vi "EXAMPLE - Determine Clicked Array Element Index.vi"() -> ()   [LabVIEW 2016]
doc: "EXAMPLE - Determine Clicked Array Element Index.vi\n\nDescription:\nThis example VI deomonstrates how to use the Determine Clicked Array Element Index VI to determine the index of the array element clicked by a user.\n\nThe VI returns the correct index whether:\n- the array is a 1D or 2D array\n- the array is displayed horizontally or vertically\n- the array label, caption, scrollbars or index display are visible or not\n- the array has an element gap displayed\n- the array array elements are physically large or small\n- the user has scrolled the visible portion of the array using either the index controls or the scrollbars\n\nNOTE: Proper operation of the Determine Clicked Array Element Index VI requires that a caption has been created for the array of interest by following the numbered steps below:\n\n(1) Right click on the array of interest and select Visible Items >> Caption\n(The item should be checked)\n\n(2) Right click on the array of interest and select Visible Items >> Caption\n(The item should be un-checked)\n\n(3) Right click on the array of interest and select Visible Items >> Label\n(The item should be checked)\n\n(4) Save the VI\n\nDeveloped By:\nMark.ridgley\nMark.Ridgley_LabVIEW.Developer@comcast.net"
panel:
  in  "stop":bool
  out "Clicked Index":i32[](array[numeric])
  in  "Tab Control":T1(tab)
  out "2D Array (With element gap)":picture[][](array[picture]) caption="2D Array"
  out "2D Array":picture[][](array[picture])
  out "2D Array of Small Elements (With elemet gap)":picture[][](array[picture])
  out "2D Array of Small Elements":picture[][](array[picture])
  out "1D Array (Vertical with elemet gap)":picture[](array[picture])
  out "1D Array (Vertical)":picture[](array[picture])
  out "1D Array (Horizontal with element gap)":picture[](array[picture])
  out "1D Array (Horizontal)":picture[](array[picture])
  out "Selected Glyph":picture
  out "Array of Glyphs":picture[][](array[picture])
  out "Selected Element":string
  out "2D Array of Strings (With element gap)":string[][](array[string]) caption="2D Array"
  # "Run the VI. Click an element in any array on any tab.\n\nThe clicked index indicator will display the index of the element you clicked.\n\nThe VI returns the correct index whether:\n- the array is a 1D or 2D array\n- the array is displayed horizontally or vertically\n- the array label, caption, scrollbars or index display are visible or not\n- the array has an element gap displayed\n- the array array elements are physically large or small\n- the user has scrolled the visible portion of the array using either the index controls or the scrollbars"
  # "Row"
  # "Col"
  # "This tab demonstrates how you can use the Determine Clicked Array Element Index VI to create an interface that is similar to the glyph selector in the NI Icon Editor."
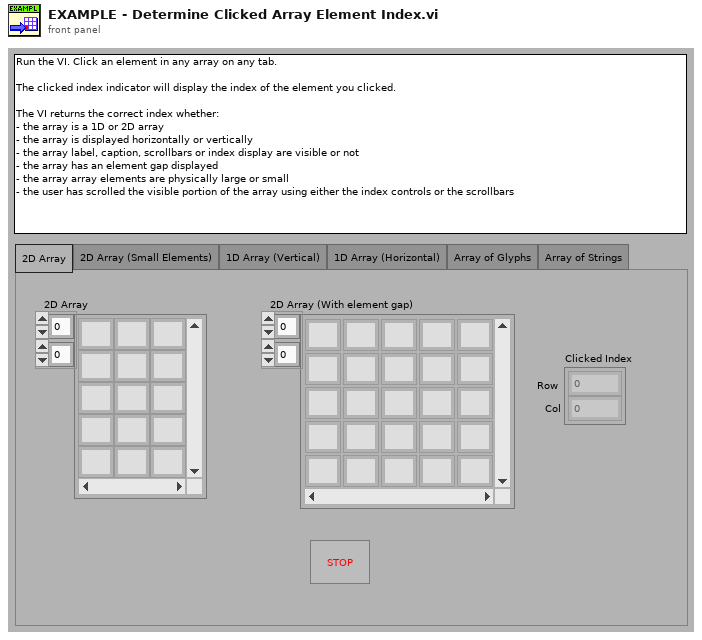
[diagram p1: front panel]
types:
  T1 = enum32{"2D Array", "2D Array (Small Elements)", "1D Array (Vertical)", "1D Array (Horizontal)", "Array of Glyphs", "Array of Strings"}
  T2 = typedef "imagedata.ctl" = cluster{"image type":i32, "image depth":i32, "image":u8[], "mask":u8[], "colors":u32[], "Rectangle":cluster{"left":i16, "top":i16, "right":i16, "bottom":i16}}
  T3 = typedef "LVPoint32TypeDef.ctl" = cluster{"Horizontal":i32, "Vertical":i32}
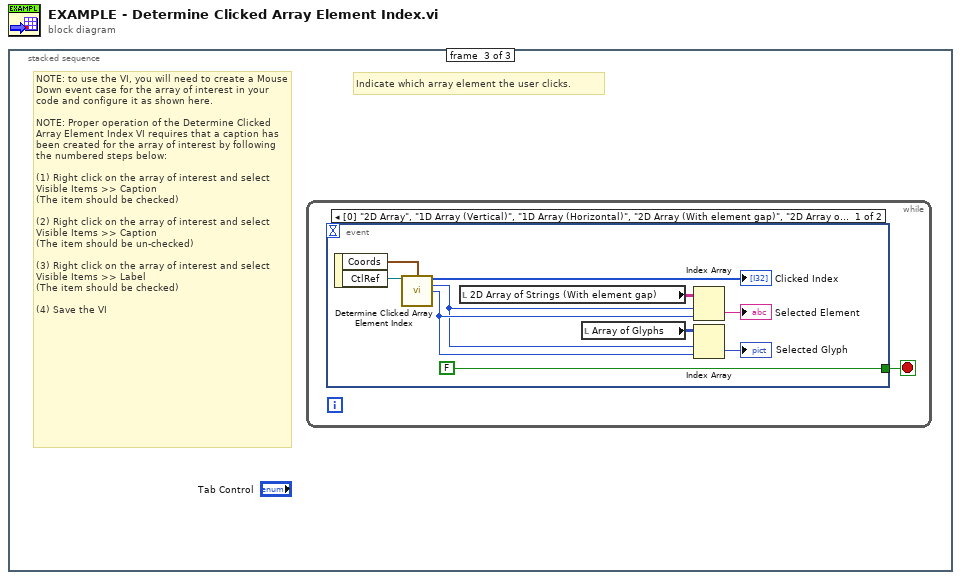
[diagram p0: block diagram]
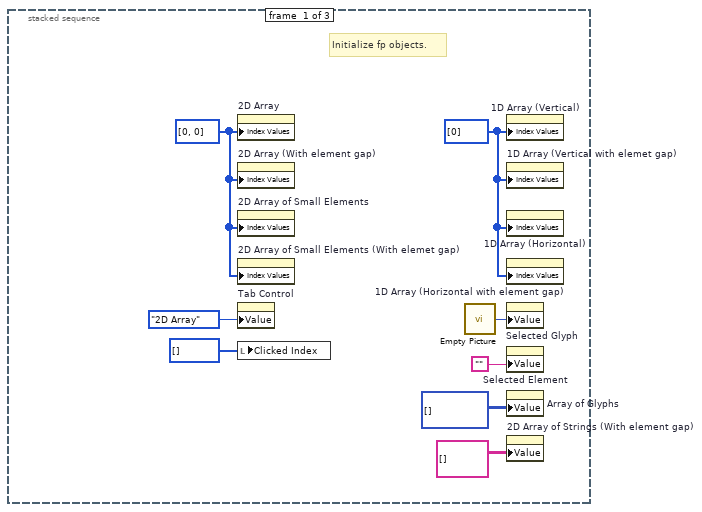
[diagram p2: hidden frame]
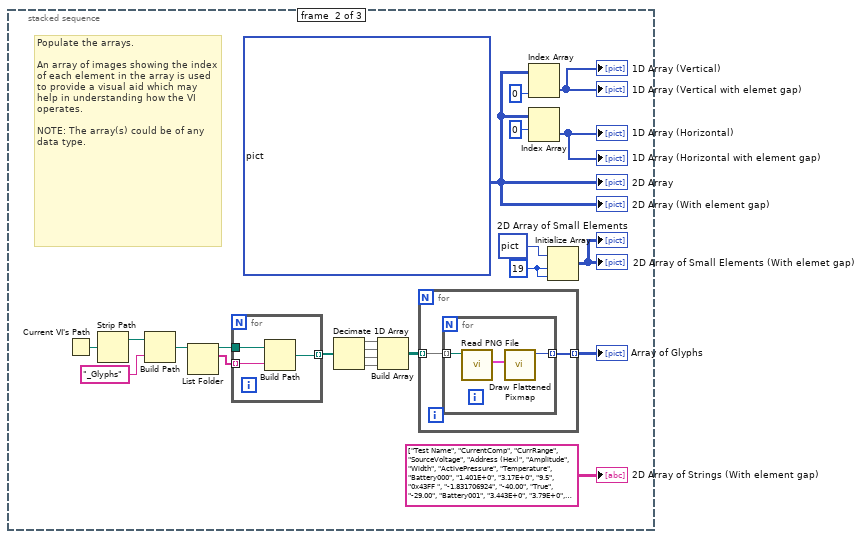
[diagram p3: hidden frame]
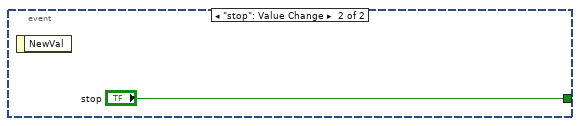
[diagram p4: hidden frame]
diagram:
  n1 = stacked-sequence {
    frame #0 {
      w6 = u32[] [0] ("Index Values")
      w7 = u32[] [0, 0] ("Selection Size[]")
      # "Initialize fp objects."
      n2 = property on="2D Array" class="Arr (strict)"("Index Values"=w7) -> ()  [unwired: 2 in, 2 out]
      n3 = property on="2D Array (With element gap)" class="Arr (strict)"("Index Values"=w7) -> ()  [unwired: 2 in, 2 out]
      n4 = property on="2D Array of Small Elements" class="Arr (strict)"("Index Values"=w7) -> ()  [unwired: 2 in, 2 out]
      n5 = property on="2D Array of Small Elements (With elemet gap)" class="Arr (strict)"("Index Values"=w7) -> ()  [unwired: 2 in, 2 out]
      n6 = property on="Tab Control" class="TabCtl (strict)"("Value"=T1."2D Array" ("Tab Control")) -> ()  [unwired: 2 in, 2 out]
      n7 = local write "Clicked Index"(i32[] [] ("Clicked Index")) -> ()
      n8 = call "Empty Picture"() -> ("empty picture"=w4:picture)
      n9 = property on="1D Array (Vertical)" class="Arr (strict)"("Index Values"=w6) -> ()  [unwired: 2 in, 2 out]
      n10 = property on="1D Array (Vertical with elemet gap)" class="Arr (strict)"("Index Values"=w6) -> ()  [unwired: 2 in, 2 out]
      n11 = property on="1D Array (Horizontal)" class="Arr (strict)"("Index Values"=w6) -> ()  [unwired: 2 in, 2 out]
      n12 = property on="1D Array (Horizontal with element gap)" class="Arr (strict)"("Index Values"=w6) -> ()  [unwired: 2 in, 2 out]
      n13 = property on="Selected Glyph" class="Pict"("Value"=w4) -> ()  [unwired: 2 in, 2 out]
      n14 = property on="Selected Element" class="Str"("Value"="") -> ()  [unwired: 2 in, 2 out]
      n15 = property on="Array of Glyphs" class="Arr (strict)"("Value"=picture[][] [] ("Array of Glyphs")) -> ()  [unwired: 2 in, 2 out]
      n16 = property on="2D Array of Strings (With element gap)" class="Arr (strict)"("Value"=string[][] [] ("2D Array of Strings (With element gap)")) -> ()  [unwired: 2 in, 2 out]
    }
    frame #1 {
      w27 = 19 ("dimension size")
      w26 = picture[][] [[bytes[3102], bytes[3102], bytes[3102], bytes[3102], bytes[3102]], [bytes[3102], bytes[3102], bytes[3102], bytes[3102], bytes[3102]], [bytes[3102], bytes[3102], bytes[3102], bytes[3102], bytes[3102]], [bytes[3102], bytes[3102], bytes[3102], bytes[3102], bytes[3102]], [bytes[3102], bytes[3102], bytes[3102], bytes[3102], bytes[3102]], [bytes[3102], bytes[3102], bytes[3102], bytes[3102], bytes[3102]], [bytes[3102], bytes[3102], bytes[3102], bytes[3102], bytes[3102]]] ("Array")
      # "Populate the arrays.\n\nAn array of images showing the index of each element in the array is used to provide a visual aid which may help in understanding how the VI operates.\n\nNOTE: The array(s) could be of any data type."
      n17 = Current VI's Path() -> (path=w10:path)
      n18 = Strip Path(path=w10) -> (stripped path=w11:path)  [unwired: 1 out]
      n19 = Build Path(base path=w11, name or relative path="_Glyphs") -> (appended path=w13:path)
      n20 = List Folder(path=w13) -> (path out=w22:path, filenames=w21:string[])  [unwired: 3 in, 2 out]
      n21 = for {
        tunnel: w22 -> [w33]
        tunnel: w21 -> [w32] mode=indexing
        tunnel: [w31] -> w20 mode=indexing
        n22 = Build Path(base path=w33, name or relative path=w32) -> (appended path=w31:path)
      }
      n23 = Decimate 1D Array(w20) -> (w19:path[], w18:path[], w17:path[], w16:path[])
      n24 = Build Array(w19, w18, w17, w16) -> (w15:path[][])
      n25 = for {
        tunnel: w15 -> [w35] mode=indexing
        tunnel: [w34] -> w14 mode=indexing
        n26 = for {
          tunnel: w35 -> [w37] mode=indexing
          tunnel: [w36] -> w34 mode=indexing
          n27 = call <vilib>:"Read PNG File.vi"("path to PNG file"=w37) -> ("image data"=w38:T2)  [unwired: 8 in, 2 out]
          n28 = call <vilib>:"Draw Flattened Pixmap.vi"("image data"=w38) -> ("new picture"=w36:picture)  [unwired: 8 in]
        }
      }
      "Array of Glyphs" <- w14
      n29 = Index Array(array=w26, index (col)=0 ("index (row)")) -> (element=→"1D Array (Vertical)" →"1D Array (Vertical with elemet gap)":picture[])  [unwired: 1 in]
      n30 = Index Array(array=w26, index (row)=0) -> (element=→"1D Array (Horizontal)" →"1D Array (Horizontal with element gap)":picture[])  [unwired: 1 in]
      n31 = Initialize Array(picture bytes[3102] ("Source Icon 2"), w27, w27) -> (→"2D Array of Small Elements" →"2D Array of Small Elements (With elemet gap)":picture[][])
      "2D Array" <- w26
      "2D Array (With element gap)" <- w26
      "2D Array of Strings (With element gap)" <- string[][] [["Test Name", "CurrentComp", "CurrRange", "SourceVoltage", "Address (Hex)", "Amplitude", "Width", "ActivePressure", "Temperature"], ["Battery000", "1.401E+0", "3.17E+0", "9.5", "0x43FF ", "-1.831706924", "-40.00", "True", "-29.00"], ["Battery001", "3.443E+0", "3.79E+0", "12", "0x7740 ", "3.258019614", "20.00", "False", "12.00"], ["Battery002", "1.234E+0", "3.79E+0", "12", "0x0896 ", "1.482121841", "10.00", "True", "1.00"], ["Battery003", "5.058E-1", "3.54E-1", "2.8", "0x7F5D ", "0.218707632", "40.00", "False", "26.00"], ["Battery004", "3.576E+0", "2.40E+0", "5.0", "0x4C5D ", "1.896321814", "50.00", "True", "33.00"], ["Battery005", "2.621E+0", "3.96E+0", "12", "0x597E ", "-3.832147003", "-50.00", "False", "-37.00"], ["Battery006", "3.412E+0", "1.21E+0", "3.2", "0x9157 ", "3.655155688", "50.00", "True", "36.00"], ["Battery007", "1.892E-1", "2.05E+0", "5.0", "0xC4F4 ", "0.418100465", "50.00", "False", "33.00"], ["Battery008", "2.545E+0", "1.76E+0", "5.0", "0x4104 ", "1.217330504", "20.00", "True", "9.00"], ["Battery009", "2.001E+0", "1.25E+0", "3.2", "0x63E6 ", "0.527299613", "40.00", "False", "27.00"], ["Battery010", "3.321E+0", "8.32E-1", "3.2", "0x1037 ", "2.886781355", "20.00", "True", "9.00"], ["Battery011", "1.465E-1", "3.86E+0", "12", "0xB6C7 ", "-2.357246211", "-50.00", "False", "-33.00"], ["Battery012", "2.640E+0", "1.96E+0", "5.0", "0x3B42 ", "2.190596301", "20.00", "True", "6.00"], ["Battery013", "2.497E+0", "2.57E+0", "9.5", "0xF93E ", "3.671957813", "20.00", "False", "10.00"], ["Battery014", "6.562E-1", "2.50E+0", "9.5", "0x2A37 ", "1.571854839", "40.00", "True", "28.00"], ["Battery015", "1.097E+0", "3.87E-1", "2.8", "0xE387 ", "-0.004756799", "-20.00", "False", "-6.00"], ["Battery016", "7.752E-1", "1.72E+0", "5.0", "0x379B ", "-0.133958890", "-40.00", "True", "-27.00"], ["Battery017", "1.462E-1", "1.36E+0", "3.2", "0x5E81 ", "0.515627474", "20.00", "False", "11.00"], ["Battery018", "2.781E+0", "2.24E+0", "5.0", "0x03C5 ", "1.558517037", "50.00", "True", "33.00"], ["Battery019", "2.611E+0", "9.25E-1", "3.2", "0x8141 ", "3.453373492", "50.00", "False", "35.00"], ["Battery020", "7.248E-1", "5.72E-1", "3.2", "0x3C7D ", "1.344536011", "40.00", "True", "26.00"], ["Battery021", "1.650E+0", "3.43E+0", "9.5", "0x3454 ", "0.440924918", "20.00", "False", "13.00"], ["Battery022", "3.005E+0", "1.93E+0", "5.0", "0x77F2 ", "2.402325507", "30.00", "True", "17.00"], ["Battery023", "3.476E+0", "2.68E+0", "9.5", "0x762B ", "3.415820054", "50.00", "False", "33.00"], ["Battery024", "2.270E+0", "3.61E+0", "12", "0x4CF8 ", "-1.744100321", "-40.00", "True", "-27.00"], ["Battery025", "7.415E-1", "1.47E+0", "3.2", "0x1975 ", "3.784917488", "20.00", "False", "13.00"], ["Battery026", "3.196E+0", "2.47E+0", "5.0", "0xD295 ", "2.599446607", "40.00", "True", "28.00"], ["Battery027", "4.261E-1", "2.35E+0", "5.0", "0x1F81 ", "0.355030387", "30.00", "False", "21.00"], ["Battery028", "4.842E-1", "1.54E+0", "5.0", "0xE919 ", "-0.309719253", "-40.00", "True", "-31.00"], ["Battery029", "3.226E-1", "3.23E+0", "9.5", "0xAE1E ", "3.923526960", "30.00", "False", "21.00"], ["Battery030", "1.235E+0", "2.65E+0", "9.5", "0xCC4D ", "1.710750502", "30.00", "True", "17.00"], ["Battery031", "2.481E+0", "3.62E+0", "12", "0x776A ", "2.639250675", "40.00", "False", "28.00"], ["Battery032", "3.138E+0", "1.62E+0", "5.0", "0x6046 ", "3.222667615", "50.00", "True", "33.00"], ["Battery033", "1.281E+0", "1.67E+0", "5.0", "0x1549 ", "1.819146492", "30.00", "False", "19.00"], ["Battery034", "3.153E+0", "2.51E+0", "9.5", "0x4DEC ", "-1.320400920", "-20.00", "True", "-12.00"], ["Battery035", "2.851E+0", "3.53E+0", "12", "0x61F2 ", "1.180328746", "50.00", "False", "36.00"], ["Battery036", "3.764E+0", "3.97E+0", "12", "0x5BD9 ", "2.523016472", "20.00", "True", "6.00"], ["Battery037", "5.071E-1", "8.27E-1", "3.2", "0xA944 ", "2.924935902", "20.00", "False", "10.00"], ["Battery038", "3.197E+0", "3.77E+0", "12", "0xC8F9 ", "3.384450259", "10.00", "True", "1.00"], ["Battery039", "2.151E-1", "2.90E+0", "9.5", "0xA6A5 ", "-2.276470914", "-30.00", "False", "-19.00"], ["Charging000", "2.719E+0", "4.49E-1", "2.8", "0xC085 ", "1.589971330", "10.00", "True", "1.00"], ["Charging001", "3.301E+0", "1.63E+0", "5.0", "0xAD34 ", "1.745287365", "10.00", "False", "3.00"], ["Charging002", "2.420E+0", "3.36E+0", "9.5", "0x230E ", "1.494001666", "20.00", "True", "10.00"], ["Charging003", "3.410E+0", "2.96E+0", "9.5", "0xBB6D ", "2.572368685", "50.00", "False", "35.00"], ["Charging004", "3.494E+0", "2.26E+0", "5.0", "0xBF9A ", "1.448412162", "20.00", "True", "10.00"], ["Charging005", "1.411E+0", "2.03E+0", "5.0", "0x5762 ", "1.801601416", "40.00", "False", "24.00"], ["Charging006", "2.913E-1", "1.39E+0", "3.2", "0xAD3D ", "0.931940520", "20.00", "True", "6.00"], ["Charging007", "3.774E+0", "3.66E+0", "12", "0x6ABF ", "0.752979651", "20.00", "False", "10.00"], ["Charging008", "3.281E+0", "1.61E+0", "5.0", "0x4C08 ", "1.738068139", "40.00", "True", "24.00"], ["Charging009", "9.122E-1", "3.36E+0", "9.5", "0x3B01 ", "2.625829738", "50.00", "False", "33.00"], ["Charging010", "3.343E-1", "2.46E+0", "5.0", "0xFDE7 ", "0.612548293", "40.00", "True", "30.00"], ["Charging011", "9.293E-1", "2.02E+0", "5.0", "0xFEFE ", "1.419903675", "10.00", "False", "2.00"], ["Charging012", "3.791E+0", "3.66E+0", "12", "0xE94A ", "-0.173060672", "-20.00", "True", "-6.00"], ["Charging013", "1.785E+0", "3.08E+0", "9.5", "0x4839 ", "-1.954966736", "-30.00", "False", "-14.00"], ["Charging014", "2.095E-1", "9.85E-1", "3.2", "0x33E0 ", "-0.838450423", "-40.00", "True", "-24.00"], ["Charging015", "1.739E+0", "1.39E+0", "3.2", "0xF318 ", "2.816093848", "40.00", "False", "28.00"], ["Charging016", "1.950E+0", "2.20E+0", "5.0", "0x8D26 ", "-1.985549142", "-50.00", "True", "-36.00"], ["Charging017", "9.482E-1", "3.46E+0", "9.5", "0xD294 ", "-2.855929041", "-20.00", "False", "-8.00"], ["Charging018", "2.719E+0", "1.30E-1", "2.8", "0x4C9F ", "2.633742761", "40.00", "True", "26.00"], ["Charging019", "1.305E+0", "2.26E+0", "5.0", "0xB04F ", "0.432901111", "50.00", "False", "36.00"], ["Charging020", "2.811E+0", "7.85E-1", "3.2", "0x40D1 ", "-0.339733120", "-40.00", "True", "-26.00"], ["Charging021", "1.089E-1", "2.17E+0", "5.0", "0x9DE1 ", "2.488760244", "20.00", "False", "11.00"], ["Charging022", "1.429E+0", "1.72E+0", "5.0", "0x611F ", "1.536641194", "50.00", "True", "36.00"], ["Charging023", "1.097E+0", "6.05E-1", "3.2", "0x3AD9 ", "0.462229914", "40.00", "False", "26.00"], ["Charging024", "3.485E+0", "1.07E+0", "3.2", "0xC999 ", "0.657049648", "30.00", "True", "18.00"], ["Charging025", "2.947E+0", "2.69E+0", "9.5", "0xED45 ", "-0.769743538", "-20.00", "False", "-5.00"], ["Charging026", "1.678E+0", "2.84E+0", "9.5", "0x51AA ", "1.226095865", "20.00", "True", "6.00"], ["Charging027", "1.273E+0", "3.32E+0", "9.5", "0xEC34 ", "-0.067737001", "-20.00", "False", "-7.00"], ["Charging028", "3.577E+0", "4.74E-1", "2.8", "0x1CFD ", "-3.647900786", "-10.00", "True", "-4.00"], ["Charging029", "2.076E+0", "2.77E+0", "9.5", "0x0D93 ", "1.714576726", "10.00", "False", "2.00"], ["Charging030", "4.247E-1", "3.10E-1", "2.8", "0x7C0C ", "2.141836453", "50.00", "True", "36.00"], ["Charging031", "2.907E-1", "1.04E+0", "3.2", "0x5A75 ", "-2.506333733", "-40.00", "False", "-27.00"], ["Charging032", "3.813E-1", "2.44E+0", "5.0", "0xAC25 ", "-3.786644694", "-30.00", "True", "-18.00"], ["Charging033", "2.421E+0", "1.46E+0", "3.2", "0xD012 ", "1.880266617", "20.00", "False", "12.00"], ["Charging034", "3.786E+0", "2.30E+0", "5.0", "0xA846 ", "1.446810509", "30.00", "True", "14.00"], ["Charging035", "1.299E+0", "3.06E+0", "9.5", "0xC7D2 ", "0.402160189", "40.00", "False", "29.00"], ["Charging036", "3.620E+0", "1.50E+0", "3.2", "0x37BE ", "1.493406399", "40.00", "True", "26.00"], ["Charging037", "7.669E-1", "2.78E+0", "9.5", "0x8857 ", "-2.239893819", "-50.00", "False", "-35.00"], ["Charging038", "1.831E+0", "3.21E+0", "9.5", "0x2AFA ", "1.499815472", "40.00", "True", "29.00"], ["Charging039", "2.502E+0", "1.53E+0", "5.0", "0x8432 ", "1.168645429", "30.00", "False", "17.00"], ["Response000", "2.017E+0", "2.52E+0", "9.5", "0xF3A2 ", "-3.391803411", "-10.00", "True", "-1.00"], ["Response001", "1.621E+0", "1.48E+0", "3.2", "0x9095 ", "1.433574608", "20.00", "False", "14.00"], ["Response002", "2.145E+0", "3.10E+0", "9.5", "0x07B9 ", "-1.536879618", "-40.00", "True", "-31.00"], ["Response003", "2.086E+0", "3.53E+0", "12", "0x3F8E ", "1.116298173", "40.00", "False", "25.00"], ["Response004", "2.024E+0", "2.91E+0", "9.5", "0x681C ", "0.891619051", "20.00", "True", "10.00"], ["Response005", "2.314E+0", "2.51E+0", "9.5", "0xD1D1 ", "1.058995824", "30.00", "False", "21.00"], ["Response006", "1.545E+0", "2.91E+0", "9.5", "0xECC2 ", "0.176933101", "20.00", "True", "5.00"], ["Response007", "2.060E+0", "2.24E-1", "2.8", "0x755D ", "-0.456950105", "-20.00", "False", "-5.00"], ["Response008", "2.116E+0", "3.85E+0", "12", "0xA85B ", "2.967945105", "40.00", "True", "26.00"], ["Response009", "3.801E+0", "1.66E+0", "5.0", "0x72B9 ", "-2.559504517", "-20.00", "False", "-12.00"], ["Response010", "7.085E-2", "5.27E-1", "3.2", "0x7A14 ", "-3.745907159", "-10.00", "True", "-4.00"], ["Response011", "8.132E-1", "1.26E+0", "3.2", "0x8F3C ", "1.040024088", "50.00", "False", "35.00"], ["Response012", "3.044E-1", "1.60E+0", "5.0", "0xBCCE ", "0.031241333", "20.00", "True", "8.00"], ["Response013", "2.818E+0", "2.58E+0", "9.5", "0x1B52 ", "-0.666424901", "-50.00", "False", "-34.00"], ["Response014", "3.028E+0", "2.67E+0", "9.5", "0x73AE ", "-3.366652376", "-40.00", "True", "-27.00"], ["Response015", "1.615E+0", "3.37E+0", "9.5", "0xDE40 ", "-2.883032187", "-40.00", "False", "-29.00"], ["Response016", "1.842E+0", "2.64E+0", "9.5", "0xAC24 ", "-0.677554620", "-20.00", "True", "-7.00"], ["Response017", "2.004E+0", "2.64E+0", "9.5", "0x89AE ", "2.782365515", "20.00", "False", "13.00"], ["Response018", "2.395E+0", "1.04E+0", "3.2", "0xE2CF ", "3.160972349", "40.00", "True", "28.00"], ["Response019", "2.227E+0", "3.64E+0", "12", "0xE55D ", "-3.111005601", "-10.00", "False", "-4.00"], ["Response020", "3.513E+0", "1.98E+0", "5.0", "0x2DBF ", "-3.997677418", "-20.00", "True", "-13.00"], ["Response021", "2.436E+0", "2.98E+0", "9.5", "0x6B36 ", "-3.358214850", "-50.00", "False", "-35.00"], ["Response022", "9.235E-1", "1.11E+0", "3.2", "0x01DD ", "2.953338993", "40.00", "True", "25.00"], ["Response023", "1.670E+0", "2.07E+0", "5.0", "0x5170 ", "0.737676437", "20.00", "False", "13.00"], ["Response024", "1.601E+0", "8.70E-1", "3.2", "0x66B0 ", "2.202349878", "10.00", "True", "3.00"], ["Response025", "2.798E+0", "4.06E-1", "2.8", "0x863A ", "0.453691159", "30.00", "False", "16.00"], ["Response026", "5.829E-1", "3.50E+0", "12", "0x19BC ", "1.899301739", "30.00", "True", "22.00"], ["Response027", "1.977E+0", "2.43E+0", "5.0", "0xAB8A ", "1.129472282", "40.00", "False", "23.00"], ["Response028", "3.446E+0", "3.07E+0", "9.5", "0x679B ", "2.815345821", "20.00", "True", "10.00"], ["Response029", "1.695E+0", "3.57E+0", "12", "0xEB27 ", "1.371177703", "40.00", "False", "26.00"], ["Response030", "1.392E+0", "8.82E-1", "3.2", "0x3EF0 ", "-2.238957936", "-30.00", "True", "-22.00"], ["Response031", "2.927E+0", "1.61E+0", "5.0", "0x7DF4 ", "3.854720233", "10.00", "False", "1.00"], ["Response032", "2.465E+0", "3.91E+0", "12", "0xAFC3 ", "-2.965422089", "-40.00", "True", "-26.00"], ["Response033", "3.533E-1", "3.75E+0", "12", "0x48C5 ", "0.733472542", "50.00", "False", "35.00"], ["Response034", "4.270E-1", "1.01E+0", "3.2", "0xD3C4 ", "2.870952249", "10.00", "True", "2.00"], ["Response035", "2.272E+0", "1.57E-1", "2.8", "0x6954 ", "0.179777171", "20.00", "False", "8.00"], ["Response036", "3.889E+0", "1.44E+0", "3.2", "0x1DD4 ", "-2.602164689", "-10.00", "True", "-0.00"], ["Response037", "2.486E+0", "6.17E-1", "3.2", "0xF3B0 ", "0.580553882", "40.00", "False", "32.00"], ["Response038", "3.653E+0", "4.23E-1", "2.8", "0xD0DF ", "3.781332036", "40.00", "True", "29.00"], ["Response039", "2.917E+0", "4.26E-1", "2.8", "0x09D5 ", "0.006190673", "20.00", "False", "6.00"], ["Video000", "2.984E+0", "3.83E+0", "12", "0xA9E3 ", "1.796896605", "40.00", "True", "27.00"], ["Video001", "3.739E+0", "3.49E+0", "9.5", "0x1FEE ", "-2.180669306", "-20.00", "False", "-10.00"], ["Video002", "1.748E+0", "1.70E+0", "5.0", "0xF226 ", "0.931520707", "10.00", "True", "2.00"], ["Video003", "8.945E-2", "9.35E-1", "3.2", "0x0CDA ", "0.098854323", "40.00", "False", "24.00"], ["Video004", "3.989E+0", "2.71E+0", "9.5", "0x2854 ", "-1.608354893", "-30.00", "True", "-16.00"], ["Video005", "2.649E-1", "1.76E-1", "2.8", "0x5B9C ", "2.184460878", "50.00", "False", "35.00"], ["Video006", "3.976E+0", "4.76E-1", "2.8", "0xD0DB ", "-0.092203461", "-30.00", "True", "-20.00"], ["Video007", "8.357E-1", "8.74E-1", "3.2", "0xDE4F ", "0.820645414", "30.00", "False", "14.00"], ["Video008", "9.117E-1", "1.71E+0", "5.0", "0x8B09 ", "-0.485497006", "-40.00", "True", "-31.00"], ["Video009", "1.947E+0", "2.63E+0", "9.5", "0x8EFB ", "1.397978567", "40.00", "False", "26.00"], ["Video010", "1.995E-1", "3.35E-1", "2.8", "0xBAC9 ", "0.288882061", "50.00", "True", "36.00"], ["Video011", "3.096E+0", "1.99E+0", "5.0", "0xB80B ", "3.168643594", "20.00", "False", "13.00"], ["Video012", "3.348E+0", "1.93E+0", "5.0", "0xC56B ", "-0.953741401", "-20.00", "True", "-5.00"], ["Video013", "3.407E+0", "3.12E+0", "9.5", "0x29D0 ", "-3.377704218", "-30.00", "False", "-17.00"], ["Video014", "9.296E-1", "3.32E+0", "9.5", "0xE02B ", "1.376990718", "30.00", "True", "20.00"], ["Video015", "2.181E+0", "1.18E+0", "3.2", "0xEC05 ", "-0.581518644", "-40.00", "False", "-28.00"], ["Video016", "3.910E+0", "1.28E+0", "3.2", "0xD95D ", "2.137188058", "30.00", "True", "17.00"], ["Video017", "1.996E+0", "9.56E-1", "3.2", "0x26B0 ", "-1.070613480", "-20.00", "False", "-8.00"], ["Video018", "3.270E+0", "2.42E+0", "5.0", "0x3397 ", "-3.293521751", "-20.00", "True", "-5.00"], ["Video019", "8.340E-1", "2.30E+0", "5.0", "0x8A6A ", "2.996315968", "40.00", "False", "31.00"], ["Video020", "7.347E-1", "2.80E+0", "9.5", "0xD1C2 ", "-1.018862474", "-40.00", "True", "-24.00"], ["Video021", "1.316E+0", "1.54E+0", "5.0", "0x3647 ", "-0.343189188", "-20.00", "False", "-6.00"], ["Video022", "3.282E+0", "5.30E-1", "3.2", "0x0CB8 ", "-3.095555809", "-40.00", "True", "-27.00"], ["Video023", "3.168E-1", "3.36E+0", "9.5", "0x4DD6 ", "3.904347854", "30.00", "False", "15.00"], ["Video024", "1.723E+0", "1.71E+0", "5.0", "0x784A ", "2.251210128", "40.00", "True", "24.00"], ["Video025", "3.865E+0", "5.96E-1", "3.2", "0x1F61 ", "0.533830947", "20.00", "False", "9.00"], ["Video026", "3.281E+0", "3.06E+0", "9.5", "0x94BC ", "-0.646469058", "-20.00", "True", "-13.00"], ["Video027", "1.644E+0", "3.06E+0", "9.5", "0x7512 ", "3.610451989", "50.00", "False", "35.00"], ["Video028", "3.262E+0", "2.09E+0", "5.0", "0x0B88 ", "2.688988373", "40.00", "True", "30.00"], ["Video029", "2.175E+0", "3.58E-1", "2.8", "0xDF7D ", "2.530065076", "20.00", "False", "7.00"], ["Video030", "2.985E+0", "6.40E-1", "3.2", "0x132F ", "-2.849666705", "-40.00", "True", "-31.00"], ["Video031", "9.472E-1", "3.15E+0", "9.5", "0xF545 ", "0.934166148", "20.00", "False", "5.00"], ["Video032", "4.003E-1", "3.89E-2", "2.8", "0x4AFA ", "3.349554208", "40.00", "True", "26.00"], ["Video033", "2.737E+0", "9.07E-1", "3.2", "0xDB0C ", "-2.912199781", "-40.00", "False", "-27.00"], ["Video034", "4.603E-1", "3.42E+0", "9.5", "0x5E88 ", "0.471891428", "20.00", "True", "9.00"], ["Video035", "2.841E+0", "2.44E+0", "5.0", "0x684E ", "3.112002585", "20.00", "False", "8.00"], ["Video036", "4.245E-1", "1.79E+0", "5.0", "0xE9FE ", "0.589948421", "30.00", "True", "20.00"], ["Video037", "2.343E-1", "3.09E+0", "9.5", "0x09BF ", "-3.570733148", "-40.00", "False", "-23.00"], ["Video038", "3.003E+0", "2.22E+0", "5.0", "0x2283 ", "1.734337113", "40.00", "True", "26.00"], ["Video039", "9.848E-1", "1.45E+0", "3.2", "0xF6D1 ", "-3.565545403", "-20.00", "False", "-7.00"], ["Audio000", "2.823E+0", "3.98E+0", "12", "0x0D2B ", "-2.171562846", "-20.00", "True", "-7.00"], ["Audio001", "3.011E+0", "9.55E-1", "3.2", "0xA1E0 ", "0.174677735", "40.00", "False", "31.00"], ["Audio002", "3.069E+0", "2.89E+0", "9.5", "0x34C5 ", "-1.411127221", "-40.00", "True", "-30.00"], ["Audio003", "2.733E+0", "2.52E+0", "9.5", "0x83FF ", "-1.919275670", "-50.00", "False", "-35.00"], ["Audio004", "2.646E+0", "1.24E+0", "3.2", "0xE37B ", "-1.349953022", "-50.00", "True", "-35.00"], ["Audio005", "3.331E+0", "1.40E+0", "3.2", "0x2673 ", "2.376147984", "30.00", "False", "22.00"], ["Audio006", "2.998E+0", "4.30E-1", "2.8", "0x9D4D ", "-1.504237203", "-50.00", "True", "-36.00"], ["Audio007", "5.683E-1", "1.53E+0", "5.0", "0x3A75 ", "2.328529920", "20.00", "False", "8.00"], ["Audio008", "3.395E+0", "2.40E-1", "2.8", "0xC653 ", "2.806652390", "20.00", "True", "6.00"], ["Audio009", "2.689E+0", "3.73E+0", "12", "0x4D60 ", "2.695903371", "20.00", "False", "7.00"], ["Audio010", "2.595E+0", "2.03E-1", "2.8", "0xCD30 ", "0.578707999", "50.00", "True", "36.00"], ["Audio011", "2.032E+0", "8.02E-1", "3.2", "0x8C67 ", "1.058426759", "50.00", "False", "33.00"], ["Audio012", "2.768E+0", "1.56E+0", "5.0", "0x5343 ", "2.239670144", "20.00", "True", "14.00"], ["Audio013", "2.932E-1", "3.68E+0", "12", "0xA5BF ", "0.781412096", "20.00", "False", "11.00"], ["Audio014", "1.141E+0", "5.54E-1", "3.2", "0x0FB4 ", "-0.652751162", "-40.00", "True", "-30.00"], ["Audio015", "5.731E-1", "1.84E+0", "5.0", "0xA25F ", "0.136921407", "40.00", "False", "30.00"], ["Audio016", "1.608E+0", "1.91E+0", "5.0", "0xB573 ", "1.339242034", "20.00", "True", "12.00"], ["Audio017", "5.658E-1", "2.03E+0", "5.0", "0x66B9 ", "1.930849604", "20.00", "False", "6.00"], ["Audio018", "4.042E-1", "3.29E+0", "9.5", "0xC505 ", "-2.049175074", "-40.00", "True", "-32.00"], ["Audio019", "2.292E+0", "2.59E+0", "9.5", "0x2CAD ", "0.977320809", "30.00", "False", "17.00"], ["Audio020", "3.499E+0", "4.78E-1", "2.8", "0x4E5B ", "0.882034848", "30.00", "True", "17.00"], ["Audio021", "1.670E+0", "8.63E-2", "2.8", "0xFBF8 ", "1.286781082", "40.00", "False", "31.00"], ["Audio022", "1.109E+0", "3.96E+0", "12", "0x57E9 ", "1.397229946", "40.00", "True", "28.00"], ["Audio023", "2.952E+0", "2.16E-1", "2.8", "0x4439 ", "-3.288879984", "-30.00", "False", "-18.00"], ["Audio024", "1.536E+0", "2.23E+0", "5.0", "0x2567 ", "-0.268866376", "-30.00", "True", "-23.00"], ["Audio025", "2.667E+0", "3.66E-3", "2.8", "0x9938 ", "0.418220053", "20.00", "False", "14.00"], ["Audio026", "2.783E+0", "6.66E-1", "3.2", "0xE58F ", "0.527376640", "10.00", "True", "2.00"], ["Audio027", "4.279E-1", "6.90E-3", "2.8", "0xCD50 ", "2.081360454", "30.00", "False", "16.00"], ["Audio028", "1.548E+0", "8.73E-1", "3.2", "0xD4A4 ", "2.197037408", "10.00", "True", "1.00"], ["Audio029", "1.166E+0", "2.06E+0", "5.0", "0xF48A ", "2.273049528", "40.00", "False", "23.00"], ["Audio030", "1.069E+0", "4.21E-1", "2.8", "0x7DED ", "3.084104251", "20.00", "True", "8.00"], ["Audio031", "3.820E+0", "1.86E+0", "5.0", "0x5226 ", "0.613830657", "40.00", "False", "25.00"], ["Audio032", "2.275E+0", "3.05E+0", "9.5", "0x492D ", "-1.661684300", "-20.00", "True", "-14.00"], ["Audio033", "2.412E+0", "2.08E-1", "2.8", "0x727B ", "-2.611466043", "-40.00", "False", "-27.00"], ["Audio034", "3.683E+0", "4.26E-1", "2.8", "0xE191 ", "3.249593536", "10.00", "True", "4.00"], ["Audio035", "2.745E+0", "2.52E-1", "2.8", "0xBC2F ", "-3.983409564", "-10.00", "False", "-4.00"], ["Audio036", "1.872E+0", "1.68E+0", "5.0", "0x3858 ", "1.319671581", "20.00", "True", "9.00"], ["Audio037", "1.016E+0", "1.89E+0", "5.0", "0xE834 ", "2.001412204", "20.00", "False", "12.00"], ["Audio038", "3.628E+0", "4.10E-2", "2.8", "0x38C8 ", "1.652382898", "10.00", "True", "3.00"], ["Audio039", "2.554E+0", "3.35E+0", "9.5", "0x73F3 ", "-2.484625639", "-30.00", "False", "-15.00"]] ("Auto-Generated Array To Sort")
    }
    frame #2 {
      # "NOTE: to use the VI, you will need to create a Mouse Down event case for the array of interest in your code and configure it as shown here.\n\nNOTE: Proper operation of the Determine Clicked Array Element Index VI requires that a caption has been created for the array of interest by following the numbered steps below:\n\n(1) Right click on the array of interest and select Visible Items >> Caption\n(The item should be checked)\n\n(2) Right click on the array of interest and select Visible Items >> Caption\n(The item should be un-checked)\n\n(3) Right click on the array of interest and select Visible Items >> Label\n(The item should be checked)\n\n(4) Save the VI"
      # "Indicate which array element the user clicks."
      n32 = while {
        stop <- w39 stop-if-true
        n33 = event shown="[0] \"2D Array\", \"1D Array (Vertical)\", \"1D Array (Horizontal)\", \"2D Array (With element gap)\", \"2D Array of Small Elements\", \"2D Array of Small Elements (With elemet gap)\", \"1D Array (Vertical with elemet gap)\", \"1D Array (Horizontal with element gap)\", \"Array of Glyphs\", \"2D Array of Strings (With element gap)\": Mouse Down" {
          selector: _ -> [_ _]
          dyn-events: _ -> [_ _]
          timeout: _ -> [_ _]
          tunnel: [FALSE ("stop") "stop"] -> w39
          event "2D Array", "1D Array (Vertical)", "1D Array (Horizontal)", "2D Array (With element gap)", "2D Array of Small Elements", "2D Array of Small Elements (With elemet gap)", "1D Array (Vertical with elemet gap)", "1D Array (Horizontal with element gap)", "Array of Glyphs", "2D Array of Strings (With element gap)": Mouse Down {
            n34 = event-data() -> ("Coords"=w48:T3, "CtlRef"=w47:refnum<vi>)  [unwired: 1 out]
            n35 = call "Determine Clicked Array Element Index.vi"("reference"=w47, "Coords of Click"=w48) -> ("Clicked Index"=→"Clicked Index":i32[], "Clicked Row"=w42:i32, "Clicked Col"=w43:i32)  [unwired: 8 in, 3 out]
            n36 = local read "2D Array of Strings (With element gap)"() -> (w41:string[][])
            n37 = local read "Array of Glyphs"() -> (w45:picture[][])
            n38 = Index Array(array=w41, index (row)=w42, index (col)=w43) -> (element=→"Selected Element":string)
            n39 = Index Array(array=w45, index (row)=w42, index (col)=w43) -> (element=→"Selected Glyph":picture)
          }
          event "stop": Value Change {
            n40 = event-data() -> ()  [unwired: 2 out]
          }
        }
      }
    }
  }
